vi "DESTROY UE.vi"(8 "error in (no error)":errorcluster, 11 "GUARDADOTEXTOPLANO in":refnum<class "GUARDADOTEXTOPLANO.lvclass">) -> (0 "error out":errorcluster, 3 "GUARDADOTEXTOPLANO out":refnum<class "GUARDADOTEXTOPLANO.lvclass">)   [LabVIEW 2019, in "GUARDADOTEXTOPLANO.lvlib" / "GUARDADOTEXTOPLANO.lvclass"]
uses:
  GUARDADOTEXTOPLANO.lvclass
  GUARDADOTEXTOPLANO.lvclass/GUARDADOTEXTOPLANO.ctl
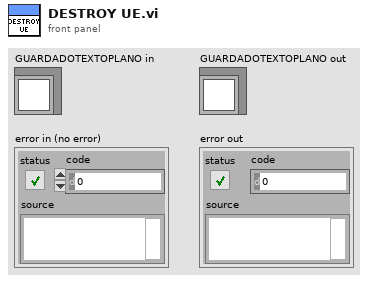
[diagram p1: front panel]
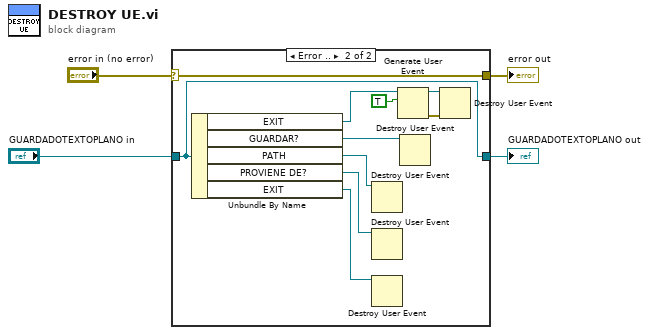
[diagram p0: block diagram]
diagram:
  n1 = case shown="Error .." "error in (no error)" {
    selector: "error in (no error)" -> [w5 w9]
    tunnel: [w6 w16] -> w3
    tunnel: "GUARDADOTEXTOPLANO in" -> [w6 w16]
    tunnel: [w5 w9] -> w4
    frame No Error {
    }
    frame Error {
      n2 = Unbundle By Name(w16) -> ("EXIT"=w15:refnum<user-event>, "GUARDAR?"=w12:refnum<user-event>, "PATH"=w11:refnum<user-event>, "PROVIENE DE?"=w10:refnum<user-event>, "EXIT"=w7:refnum<user-event>)
      n3 = Destroy User Event(user event=w11) -> ()  [unwired: 1 in, 1 out]
      n4 = Destroy User Event(user event=w10) -> ()  [unwired: 1 in, 1 out]
      n5 = Destroy User Event(user event=w7) -> ()  [unwired: 1 in, 1 out]
      n6 = Generate User Event(user event=w15, event data cluster=TRUE ("event data")) -> (user event out=w13:refnum<user-event>, error out=w14:errorcluster)  [unwired: 2 in]
      n7 = Destroy User Event(user event=w12) -> ()  [unwired: 1 in, 1 out]
      n8 = Destroy User Event(user event=w13, error in=w14) -> ()  [unwired: 1 out]
    }
  }
  "error out" <- w4
  "GUARDADOTEXTOPLANO out" <- w3
